vi "Build Email.vi"(8 "error in (no error)":errorcluster, 11 "Gmail in":refnum<class "Gmail.lvclass">) -> (0 "error out":errorcluster, 2 "Email":string, 3 "Gmail out":refnum<class "Gmail.lvclass">)   [LabVIEW 2020, in "Gmail API.lvlib" / "Gmail.lvclass"]
uses:
  Gmail.lvclass
  Gmail.lvclass/Gmail.ctl
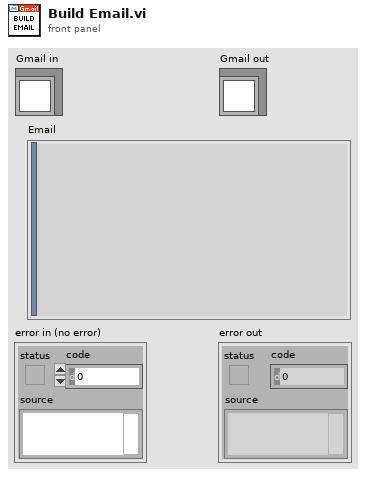
[diagram p1: front panel]
types:
  T1 = typedef "Gmail API.lvlib/Mail Address.ctl" = cluster{"Name":string, "Email":string}
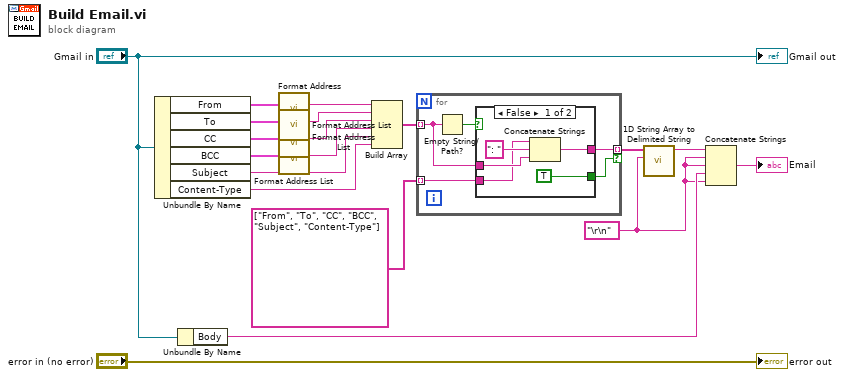
[diagram p0: block diagram]
diagram:
  w4 = "\r\n"
  n1 = Unbundle By Name("Gmail in") -> ("From"=w17:T1, "To"=w18:T1[], "CC"=w16:T1[], "BCC"=w15:T1[], "Subject"=w11:string, "Content-Type"=w10:string)
  n2 = Unbundle By Name("Gmail in") -> ("Body"=w5:string)
  n3 = call "Format Address.vi"("Address"=w17) -> ("Formatted Address"=w1:string)  [unwired: 10 in]
  n4 = call "Format Address List.vi"("Addresses"=w18) -> ("Address List"=w14:string)  [unwired: 10 in]
  n5 = call "Format Address List.vi"("Addresses"=w16) -> ("Address List"=w13:string)  [unwired: 10 in]
  n6 = call "Format Address List.vi"("Addresses"=w15) -> ("Address List"=w12:string)  [unwired: 10 in]
  n7 = Build Array(w1, w14, w13, w12, w11, w10) -> (w8:string[])
  n8 = for {
    tunnel: string[] ["From", "To", "CC", "BCC", "Subject", "Content-Type"] -> [w22] mode=indexing
    tunnel: w8 -> [w23] mode=indexing
    tunnel: [w21] -> w7 mode=indexing if=w20
    n9 = Empty String/Path?(string/path=w23) -> (empty?=w24:bool)
    n10 = case shown="False" w24 {
      tunnel: w23 -> [w26 _]
      tunnel: w22 -> [w25 _]
      tunnel: [w28 _] -> w21
      tunnel: [TRUE _] -> w20
      frame False {
        n11 = Concatenate Strings(w25, ": " ("string"), w26) -> (w28:string)
      }
      frame True {
      }
    }
  }
  n12 = call <vilib>:"1D String Array to Delimited String.vi"("delimiter"=w4, "string array"=w7) -> ("delimited string"=w6:string)  [unwired: 9 in]
  n13 = Concatenate Strings(w6, w4, w4, w5, w4) -> (→"Email":string)
  "error out" <- "error in (no error)"
  "Gmail out" <- "Gmail in"
